vi "setTemp.vi"(1 "error in (no error)":errorcluster, 2 "Heizspannung":dbl) -> (0 "error out":errorcluster)   [LabVIEW 2010]
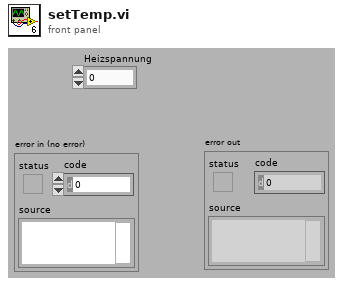
[diagram p1: front panel]
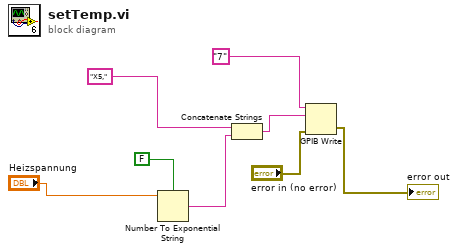
[diagram p0: block diagram]
diagram:
  n1 = Number To Exponential String(number="Heizspannung", 1:FALSE) -> (E-format string=w7:string)  [unwired: 2 in]
  n2 = Concatenate Strings("X5,", w7) -> (w5:string)
  n3 = GPIB Write(0:"7", 1:w5, 3:"error in (no error)") -> (6:→"error out":errorcluster)  [unwired: 2 in, 1 out]
